vi "Server_Demo.vi"() -> ()   [LabVIEW 2011]
uses:
  VIremote.llb/VIremoteFunction.ctl
panel:
  in  "stop":bool
  out "IP address of this computer":string
  # "If this is the first time you run this then follow the instructions below.\n\nRun This VI.\nStart VIremote on your iPhone/iPod.\nEnter the IP address of this computer (see below) on the info page. Press \"Connect\".\nThe \"Demo Input.vi\" will show on the screen. Try it out and go to next demo.\n\nView the diagram of this and all the demos to learn more.\n\nSend feedback and questions to iPhone@throwlab.com \n\n/ThrowLab"
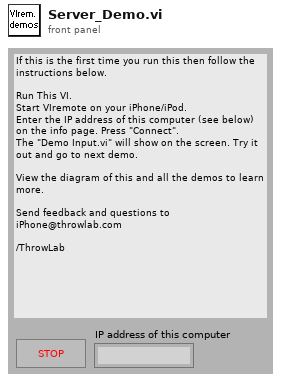
[diagram p1: front panel]
types:
  T1 = typedef "VIremoteFunction.ctl" = enum16{"Do nothing", "Stop controller", "Close this connection", "Show info panel", "Set VI to control", "Set Accelerometer freq (Hz)", "Show Alert message", "Start Sound Input", "Stop Sound Input", "Set Volume (0-100)", "Set sound output Speaker", "Set sound output Receiver", "Play Sound", "Repeat Sound", "Stop Sound", "Pause Sound", "Resume Sound", "Set panel width of caller (320 or 480)", "Set Panel Size to Portrait", "Set Panel Size to Landscape", "Set Panel Size as Current Orientation", "Allow all UI Orientations", "Send user notification", "Disable Scrolling", "Normal Scrolling", "Page Scrolling", "Set Scroll Offset", "Page Indicator Position"}
  T2 = typedef "VIremoteInit.ctl" = cluster{"port (2055)":u16, "Use mouse emulation (T)":bool, "Use keyboard emulation (T)":bool, "Allow multiple connections (F)":bool, "Debug mode/error dialog (F)":bool, "Temporary directory (default)":path, "Mouse emulation VI path":path, "Keyboard emulation VI path":path, "Enable VI Select button(T)":bool, "Enable auto scroll(T)":bool}
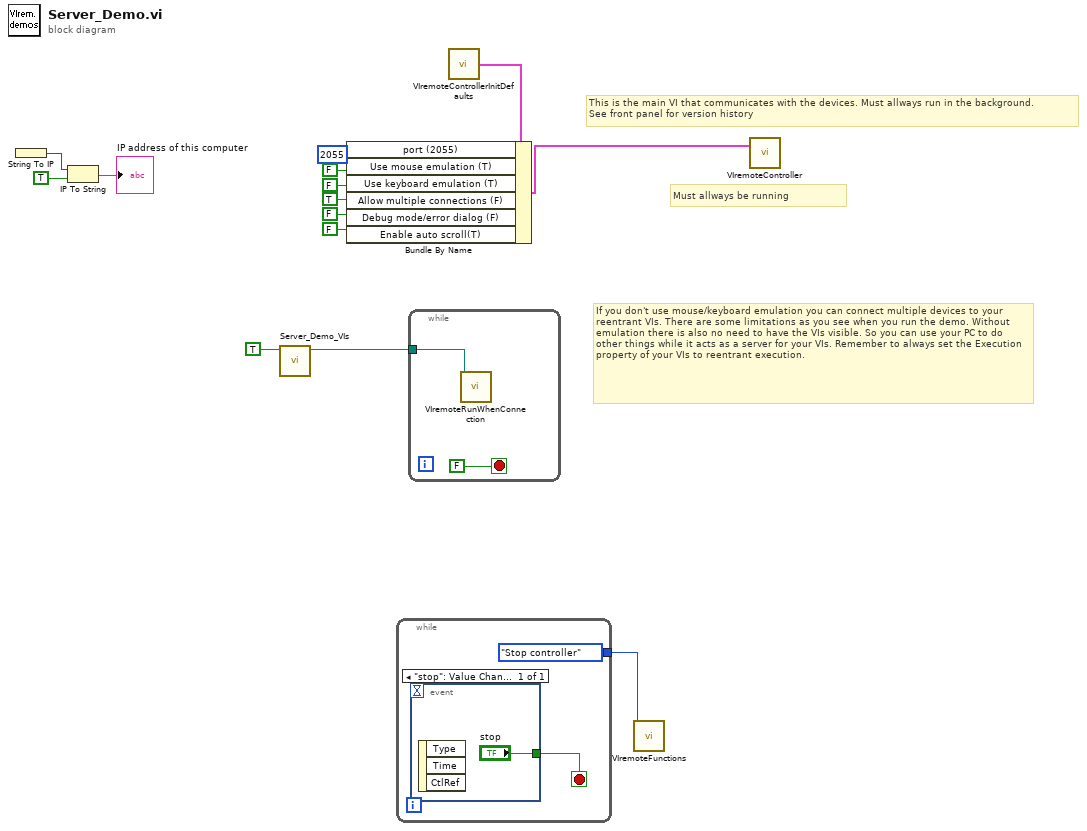
[diagram p0: block diagram]
diagram:
  # "If you don't use mouse/keyboard emulation you can connect multiple devices to your reentrant VIs. There are some limitations as you see when you run the demo. Without emulation there is also no need to have the VIs visible. So you can use your PC to do other things while it acts as a server for your VIs. Remember to always set the Execution property of your VIs to reentrant execution."
  # "Must allways be running"
  # "This is the main VI that communicates with the devices. Must allways run in the background.\nSee front panel for version history"
  n1 = String To IP() -> (0:w14:u32)  [unwired: 1 out]
  n2 = IP To String(1:TRUE ("dot notation? (F)"), 2:w14) -> (0:→"IP address of this computer":string)
  n3 = call "Server_Demo_VIs.vi"("Only get This VIs path"=TRUE) -> ("path"=w11:path)  [unwired: 10 out]
  n4 = while {
    tunnel: [VIremoteFunction."Stop controller" ("Function")] -> w4
    stop <- w16 stop-if-true
    n5 = event shown="[0] \"stop\": Value Change" {
      selector: _ -> [_]
      dyn-events: _ -> [_]
      timeout: _ -> [_]
      tunnel: ["stop"] -> w16
      event "stop": Value Change {
        n6 = event-data() -> ()  [unwired: 4 out]
      }
    }
  }
  n7 = while {
    tunnel: w11 -> [w18]
    stop <- FALSE stop-if-true
    n8 = call "VIremoteRunWhenConnection.vi"("path to VI that will be run"=w18) -> ()  [unwired: 1 in, 10 out]
  }
  n9 = call "VIremoteControllerInitDefaults.vi"() -> ("Init defaults"=w1:T2)
  n10 = Bundle By Name(cluster=w1, "port (2055)"=u16 2055, "Use mouse emulation (T)"=FALSE, "Use keyboard emulation (T)"=FALSE, "Allow multiple connections (F)"=TRUE, "Debug mode/error dialog (F)"=FALSE, "Enable auto scroll(T)"=FALSE) -> (w10:T2)
  n11 = call "VIremoteFunctions.vi"("Function"=w4) -> ()  [unwired: 5 in, 6 out]
  n12 = call "VIremoteController.vi"("Init (can't be changed while running)"=w10) -> ()  [unwired: 11 out]
